vi "TDS_ReadConfigurationFromFiles.vi"(7 "SinchronizationRefs":T1, 8 "error in":errorcluster, 11 "VI Server ClusterDUP":T3) -> (0 "error out":errorcluster)   [LabVIEW 2020]
uses:
  <vilib>/Utility/config.llb/NI_LVConfig.lvlib
  <vilib>/Utility/config.llb/Read Key (String).vi
  LabVIEW 2020 Toolkits/VI Server Toolkit/VI Server Libraries/VI Server_GetControl.llb/VI Server_ComboBox_Get.vi
  NA-E5071B/E5071B.llb/Labels&Control References.ctl
  NA-E5071B/E5071B.llb/Squib_DynamicVIs_SinchronizationRefs.ctl
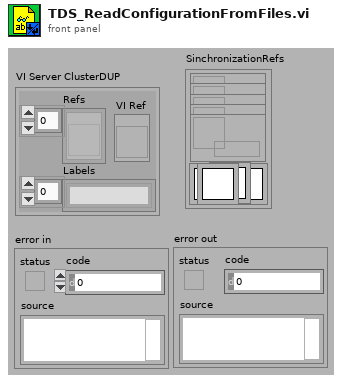
[diagram p1: front panel]
types:
  T1 = typedef "Squib_DynamicVIs_SinchronizationRefs.ctl" = cluster{"DAQmxSmaphore":T2, "InstrSemaphore":T2, "CycleEvent":refnum<notifier>, "ABORT":refnum<notifier>, "STOP":refnum<notifier>, "MessagesQ":refnum<queue>, "DMM.Measure":T2, "T&C.Write":refnum<queue>, "T&C.Read":refnum<queue>, "PM_Sinch":T2}
  T2 = typedef "Semaphore RefNum" = refnum<k1>
  T3 = typedef "Labels&Control References.ctl" = cluster{"Refs":refnum<vi>[], "Labels":string[], "VI Ref":refnum<vi>}
  T4 = typedef "VI Server_RefsCluster.ctl" = cluster{"Labels":string[], "Refs":refnum<vi>[], "VI Ref":refnum<vi>}
  T5 = typedef "NI_LVConfig.lvlib/Config Data RefNum.ctl" = refnum<k1>
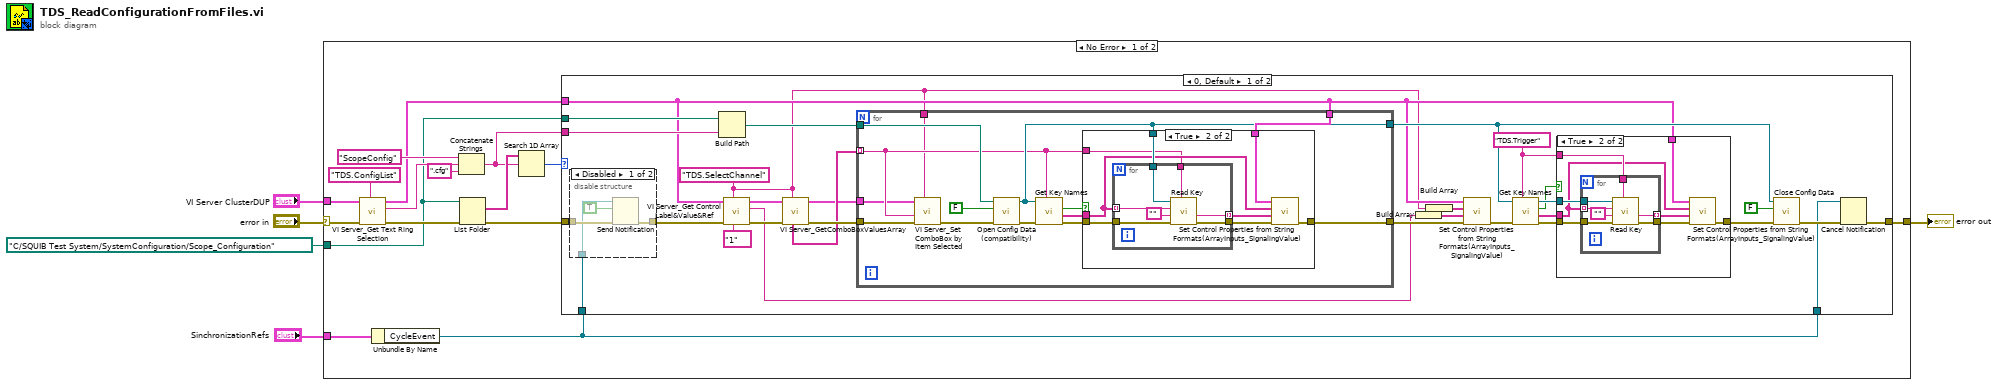
[diagram p0: block diagram]
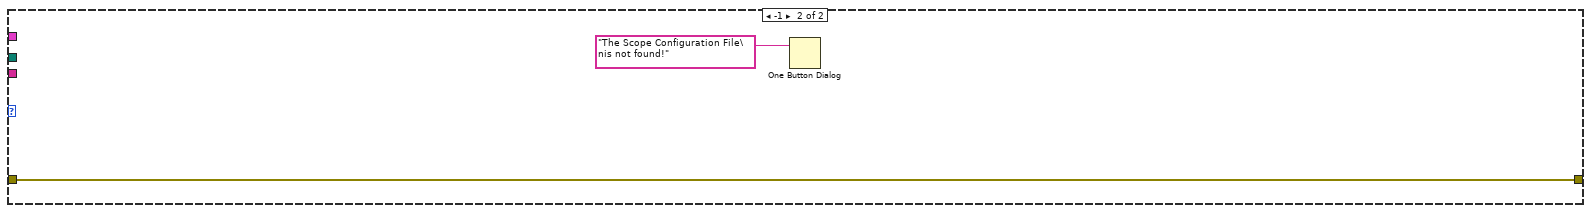
[diagram p5: hidden frame]
diagram:
  n1 = case shown="No Error" "error in" {
    selector: "error in" -> [w8 w105]
    tunnel: "VI Server ClusterDUP" -> [w15 _]
    tunnel: [w13 w105] -> w4
    tunnel: path "C:/SQUIB Test System/SystemConfiguration/Scope_Configuration" ("path") -> [w10 _]
    tunnel: "SinchronizationRefs" -> [w7 _]
    frame No Error {
      n2 = call "VI Server_Get Text Ring Selection.vi"("Label"="TDS.ConfigList", "error in"=w8, "VI Server Cluster"=w15) -> ("error out"=w20:errorcluster, "Selection"=w17:string, "VI Server dup"=w9:T3)  [unwired: 3 in, 3 out]
      n3 = Unbundle By Name(w7) -> ("CycleEvent"=w6:refnum<notifier>)
      n4 = Concatenate Strings("ScopeConfig" ("regular expression"), w17, ".cfg" ("string")) -> (w11:string)
      n5 = List Folder(path=w10, error in=w20) -> (filenames=w21:string[], error out=w14:errorcluster)  [unwired: 2 in, 2 out]
      n6 = Search 1D Array(1D array=w21, element=w11) -> (index of element=w12:i32)  [unwired: 1 in]
      n7 = case shown="0, Default" w12 {
        tunnel: w14 -> [w29 w104]
        tunnel: [w25 w104] -> w13
        tunnel: w11 -> [w51 _]
        tunnel: w10 -> [w50 _]
        tunnel: w9 -> [w34 _]
        tunnel: w6 -> [w27 _]
        tunnel: w6 -> [w24 _]
        frame 0, Default {
          w44 = "TDS.Trigger" ("section")
          w23 = "TDS.SelectChannel" ("Label")
          n8 = disable-structure shown="Disabled" {
            disable-tunnel: w29 -> [w55 w56]
            disable-tunnel: [w54 w56] -> w28
            disable-tunnel: w27 -> [w53 _]
            frame Disabled {
              n9 = Send Notification(notification=TRUE, notifier=w53, error in (no error)=w55) -> (error out=w54:errorcluster)  [unwired: 1 out]
            }
            frame Enabled {
            }
          }
          n10 = Build Path(base path=w50, name or relative path=w51) -> (appended path=w49:path)
          n11 = call-poly "VI Server_Get Control Label&Value&Ref.vi"("DataType"="1" ("Default Value"), "Control.Label"=w23, "error in"=w28, "VI Server.RefsCluster"=w34) -> ("error out"=w40:errorcluster, "Value"=w32:string, "VI Server.RefsCluster.DUP"=w38:T4)  [unwired: 4 in, 1 out]
          n12 = call <userlib>:"VI Server_GetComboBoxValuesArray.vi"("Label"=w23, "error in"=w40, "Data Cluster"=w38) -> ("error out"=w39:errorcluster, "Data Cluster dup"=w22:T3, "Values[]"=w37:string[])  [unwired: 4 in, 2 out]
          n13 = for {
            tunnel: w49 -> [w86]
            tunnel: [w84] -> w36
            tunnel: w34 -> [w83]
            tunnel: [w82] -> w41
            tunnel: w39 -> [w75]
            tunnel: w37 -> [w77] mode=indexing
            tunnel: w23 -> [w76]
            tunnel: w22 -> [w73]
            n14 = call "VI Server_Set ComboBox by Item Selected.vi"("Label"=w76, "error in"=w75, "ComboBoxValue"=w77, "Data Cluster"=w73) -> ("error out"=w74:errorcluster)  [unwired: 5 in, 2 out]
            n15 = call <vilib>:"Open Config Data (compatibility).vi"("error in (no error)"=w74, "create file if necessary (T)"=FALSE ("create file if necessary? (T)"), "configuration file path"=w86) -> ("error out"=w81:errorcluster, "refnum"=w82:T5)  [unwired: 6 in, 1 out]
            n16 = call <vilib>:"Get Key Names.vi"("section"=w77, "error in (no error)"=w81, "refnum"=w82) -> ("error out"=w80:errorcluster, "key names"=w79:string[], "section exists?"=w78:bool)  [unwired: 5 in, 1 out]
            n17 = case shown="True" w78 {
              tunnel: [w87 w94] -> w84
              tunnel: w83 -> [_ w93]
              tunnel: w82 -> [_ w92]
              tunnel: w80 -> [w87 w91]
              tunnel: w79 -> [_ w90]
              tunnel: w77 -> [_ w88]
              frame False {
              }
              frame True {
                n18 = for {
                  tunnel: [w101] -> w95
                  tunnel: w92 -> [w100]
                  tunnel: w88 -> [w99]
                  tunnel: w91 -> [w98]
                  tunnel: w90 -> [w97] mode=indexing
                  tunnel: [w96] -> w89 mode=indexing
                  n19 = call-poly <vilib>:"Read Key.vi"("section"=w99, "error in (no error)"=w98, "default value"="", "key"=w97, "refnum"=w100) -> ("error out"=w101:errorcluster, "value"=w96:string)  [unwired: 3 in, 2 out]
                }
                n20 = call "Set Control Properties from String Formats(ArrayInputs_SignalingValue).vi"("error in (no error)"=w95, "Values"=w89, "Labels"=w90, "Labels&Refs"=w93) -> ("error out"=w94:errorcluster)  [unwired: 6 in, 1 out]
              }
            }
          }
          n21 = Build Array(w32) -> (w31:string[])
          n22 = Build Array(w23) -> (w33:string[])
          n23 = call "Set Control Properties from String Formats(ArrayInputs_SignalingValue).vi"("error in (no error)"=w36, "Values"=w31, "Labels"=w33, "Labels&Refs"=w34) -> ("error out"=w35:errorcluster)  [unwired: 6 in, 1 out]
          n24 = call <vilib>:"Get Key Names.vi"("section"=w44, "error in (no error)"=w35, "refnum"=w41) -> ("error out"=w46:errorcluster, "key names"=w43:string[], "section exists?"=w30:bool, "refnum out"=w45:T5)  [unwired: 5 in]
          n25 = case shown="True" w30 {
            tunnel: w46 -> [w57 w65]
            tunnel: w45 -> [_ w64]
            tunnel: w44 -> [_ w63]
            tunnel: w43 -> [_ w62]
            tunnel: [w57 w59] -> w42
            tunnel: w34 -> [_ w58]
            frame False {
            }
            frame True {
              n26 = for {
                tunnel: w65 -> [w72]
                tunnel: [w71] -> w60
                tunnel: w64 -> [w70]
                tunnel: w63 -> [w69]
                tunnel: w62 -> [w68] mode=indexing
                tunnel: [w66] -> w61 mode=indexing
                n27 = call-poly <vilib>:"Read Key.vi"("section"=w69, "error in (no error)"=w72, "default value"="", "key"=w68, "refnum"=w70) -> ("error out"=w71:errorcluster, "value"=w66:string)  [unwired: 3 in, 2 out]
              }
              n28 = call "Set Control Properties from String Formats(ArrayInputs_SignalingValue).vi"("error in (no error)"=w60, "Values"=w61, "Labels"=w62, "Labels&Refs"=w58) -> ("error out"=w59:errorcluster)  [unwired: 6 in, 1 out]
            }
          }
          n29 = call <vilib>:"Close Config Data.vi"("error in (no error)"=w42, "write file if changed (T)"=FALSE ("write configuration file? (T)"), "refnum"=w41) -> ("error out"=w26:errorcluster)  [unwired: 7 in, 1 out]
          n30 = Cancel Notification(0:w24, 3:w26) -> (11:w25:errorcluster)  [unwired: 2 out]
        }
        frame -1 {
          n31 = One Button Dialog(message="The Scope Configuration File\nis not found!") -> ()  [unwired: 1 in, 1 out]
        }
      }
    }
    frame Error {
    }
  }
  "error out" <- w4
